vi "Print HTML Report using IE.vi"(3 "error in (no error)":errorcluster, 5 "path to HTML":string) -> (0 "error out":errorcluster)   [LabVIEW 2017, in "NI_ReportGenerationCore.lvlib"]
doc: "This VI can be used to print any document which can be opened in the Microsoft Internet Explorer."
uses:
  <vilib>/Utility/NIReport.llb/NI_ReportGenerationCore.lvlib
panel:
  in  "control":refnum<k7>(container)
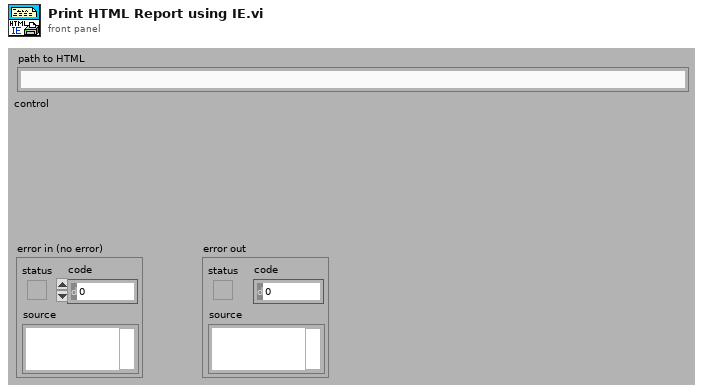
[diagram p1: front panel]
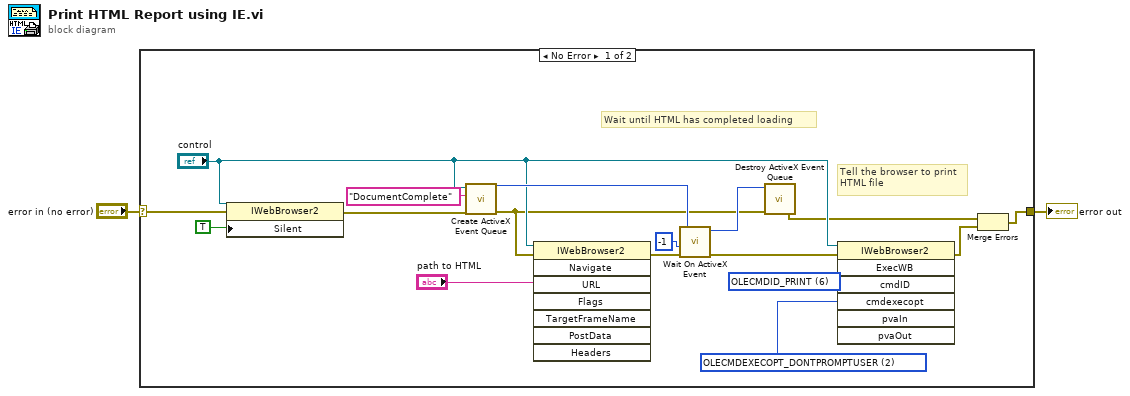
[diagram p0: block diagram]
diagram:
  n1 = case shown="No Error" "error in (no error)" {
    selector: "error in (no error)" -> [w10 w20]
    tunnel: [w3 w20] -> w1
    frame No Error {
      w18 = 2 items=["OLECMDEXECOPT_DODEFAULT", "OLECMDEXECOPT_PROMPTUSER", "OLECMDEXECOPT_DONTPROMPTUSER", "OLECMDEXECOPT_SHOWHELP"] ("cmdexecopt")
      w19 = 6 items=["OLECMDID_OPEN"=1, "OLECMDID_NEW"=2, "OLECMDID_SAVE"=3, "OLECMDID_SAVEAS"=4, "OLECMDID_SAVECOPYAS"=5, "OLECMDID_PRINT"=6, "OLECMDID_PRINTPREVIEW"=7, "OLECMDID_PAGESETUP"=8, "OLECMDID_SPELL"=9, "OLECMDID_PROPERTIES"=10, "OLECMDID_CUT"=11, "OLECMDID_COPY"=12, "OLECMDID_PASTE"=13, "OLECMDID_PASTESPECIAL"=14, "OLECMDID_UNDO"=15, "OLECMDID_REDO"=16, "OLECMDID_SELECTALL"=17, "OLECMDID_CLEARSELECTION"=18, "OLECMDID_ZOOM"=19, "OLECMDID_GETZOOMRANGE"=20, "OLECMDID_UPDATECOMMANDS"=21, "OLECMDID_REFRESH"=22, "OLECMDID_STOP"=23, "OLECMDID_HIDETOOLBARS"=24, "OLECMDID_SETPROGRESSMAX"=25, "OLECMDID_SETPROGRESSPOS"=26, "OLECMDID_SETPROGRESSTEXT"=27, "OLECMDID_SETTITLE"=28, "OLECMDID_SETDOWNLOADSTATE"=29, "OLECMDID_STOPDOWNLOAD"=30, "OLECMDID_ONTOOLBARACTIVATED"=31, "OLECMDID_FIND"=32, "OLECMDID_DELETE"=33, "OLECMDID_HTTPEQUIV"=34, "OLECMDID_HTTPEQUIV_DONE"=35, "OLECMDID_ENABLE_INTERACTION"=36, "OLECMDID_ONUNLOAD"=37, "OLECMDID_PROPERTYBAG2"=38, "OLECMDID_PREREFRESH"=39, "OLECMDID_SHOWSCRIPTERROR"=40, "OLECMDID_SHOWMESSAGE"=41, "OLECMDID_SHOWFIND"=42, "OLECMDID_SHOWPAGESETUP"=43, "OLECMDID_SHOWPRINT"=44, "OLECMDID_CLOSE"=45, "OLECMDID_ALLOWUILESSSAVEAS"=46, "OLECMDID_DONTDOWNLOADCSS"=47] ("cmdID")
      # "Tell the browser to print\nHTML file"
      # "Wait until HTML has completed loading"
      n2 = property class="IWebBrowser2"(reference="control", error in=w10, "Silent"=TRUE) -> (error out=w9:errorcluster)  [unwired: 1 out]
      n3 = call <vilib>:"Create ActiveX Event Queue.vi"("error in (no error)"=w9, "Event Name"="DocumentComplete", "Automation Refnum"="control") -> ("error out"=w7:errorcluster, "Event Queue"=w16:i32)  [unwired: 1 in, 2 out]
      n4 = invoke class="IWebBrowser2" method="Navigate"(reference="control", error in=w7, "URL"="path to HTML") -> (error out=w8:errorcluster)  [unwired: 5 in, 7 out]
      n5 = call <vilib>:"Wait On ActiveX Event.vi"("error in (no error)"=w8, "ms Timeout (-1)"=-1 ("ms timeout (-1)"), "Event Queue"=w16) -> ("error out"=w6:errorcluster, "Event Queue Out"=w15:i32)  [unwired: 1 in, 2 out]
      n6 = call <vilib>:"Destroy ActiveX Event Queue.vi"("error in (no error)"=w7, "Event Queue"=w15) -> ("error out"=w5:errorcluster)  [unwired: 5 out]
      n7 = invoke class="IWebBrowser2" method="ExecWB"(reference="control", error in=w6, "cmdID"=w19, "cmdexecopt"=w18) -> (error out=w4:errorcluster)  [unwired: 3 in, 6 out]
      n8 = Merge Errors(w5, w4) -> (w3:errorcluster)
    }
    frame Error {
    }
  }
  "error out" <- w1
